vi "AB_Log_Write_Linker.vi"(4 "destination path":path, 6 "old names":string[](array[string]), 8 "error in (no error)":errorcluster, 9 "new names":string[](array[string]), 10 "new paths":path[](array[path]), 11 "files to change":path[](array[path])) -> (0 "error out":errorcluster)   [LabVIEW 2020]
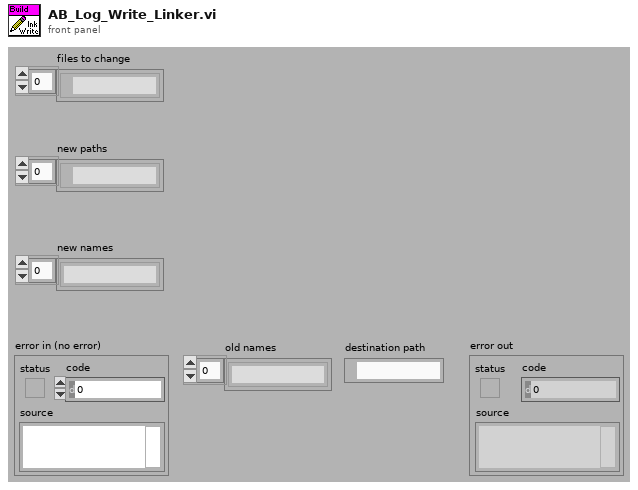
[diagram p1: front panel]
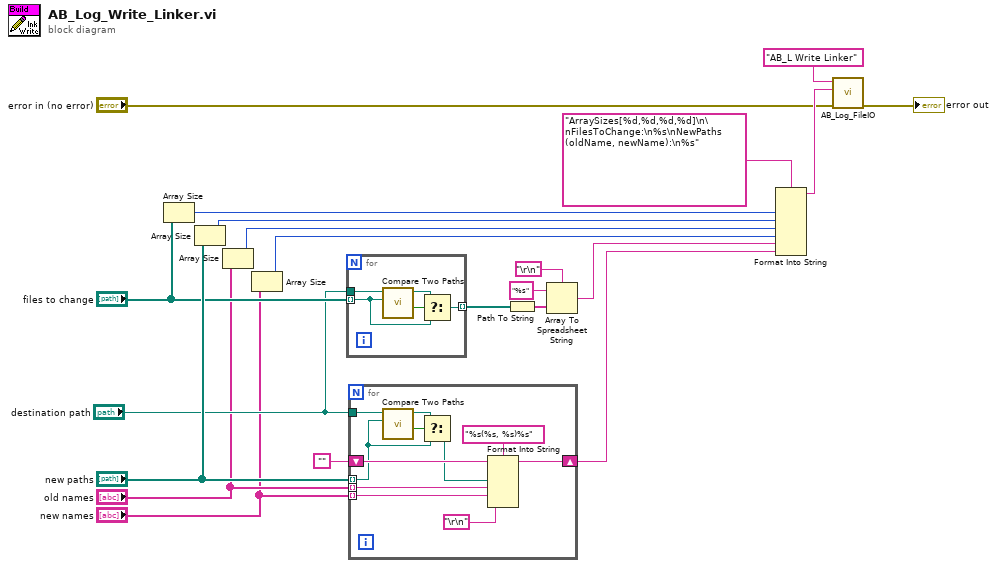
[diagram p0: block diagram]
diagram:
  n1 = Array Size(array="files to change") -> (size(s)=w11:i32)
  n2 = Array Size(array="new paths") -> (size(s)=w9:i32)
  n3 = Array Size(array="old names") -> (size(s)=w8:i32)
  n4 = Array Size(array="new names") -> (size(s)=w7:i32)
  n5 = for {
    tunnel: "files to change" -> [w24] mode=indexing
    tunnel: [w23] -> w3 mode=indexing
    tunnel: "destination path" -> [w22]
    n6 = call <vilib>:"Compare Two Paths.vi"("Path 2"=w24, "Path 1"=w22) -> ("Path 2 Relative to Path 1?"=w25:bool, "Relative Path from 1 to 2"=w26:path)  [unwired: 6 in, 2 out]
    n7 = Select(t=w26, s=w25, f=w24) -> (s? t:f=w23:path)
  }
  n8 = for {
    tunnel: "new paths" -> [w27] mode=indexing
    shift-right: [w37] -> w10
    shift-left: "" -> [w36]
    tunnel: "old names" -> [w34] mode=indexing
    tunnel: "new names" -> [w32] mode=indexing
    tunnel: "destination path" -> [w28]
    n9 = call <vilib>:"Compare Two Paths.vi"("Path 2"=w27, "Path 1"=w28) -> ("Path 2 Relative to Path 1?"=w30:bool, "Relative Path from 1 to 2"=w31:path)  [unwired: 6 in, 2 out]
    n10 = Select(t=w31, s=w30, f=w27) -> (s? t:f=w29:path)
    n11 = Format Into String(format string="%s(%s, %s)%s", initial string=w36, w29, w34, w32, "\r\n") -> (resulting string=w37:string)  [unwired: 1 in, 1 out]
  }
  n12 = Path To String(path=w3) -> (string=w14:string[])
  n13 = Array To Spreadsheet String(delimiter (Tab)="\r\n", array=w14, 3:"%s" ("format string")) -> (spreadsheet string=w12:string)
  n14 = Format Into String(format string="ArraySizes[%d,%d,%d,%d]\n\nFilesToChange:\n%s\nNewPaths (oldName, newName):\n%s", w11, w9, w8, w7, w12, w10) -> (resulting string=w20:string)  [unwired: 2 in, 1 out]
  n15 = call <vilib>:"AB_Log_FileIO.vi"("error in (no error)"="error in (no error)", "data"=w20, "newSection"="AB_L Write Linker" ("data")) -> ("error out"=→"error out":errorcluster)  [unwired: 8 in]
